vi "PolRaspPiData.vi"(8 "error in (no error)":errorcluster, 11 "VISA Sesssion In":refnum<visa-resource-name>="ASRL6::INSTR") -> (0 "error out":errorcluster, 2 "output array":string[](array[string]), 3 "VISA Sesssion Out":refnum<visa-resource-name>)   [LabVIEW 2019]
panel:
  # "The intention of this is to connect to a raspberry pi and ping for data with either 'Ping' or a number.\nThe intention of this structure is to establish modbus communication. The cRIO cannot acheive this for some reason.\nThe raspPi will monitor the furnace and heatrope data.\nIt will eventually set the furnace setpoint too (later down the line).\n\nThis assumes the serial channel has already been opened"
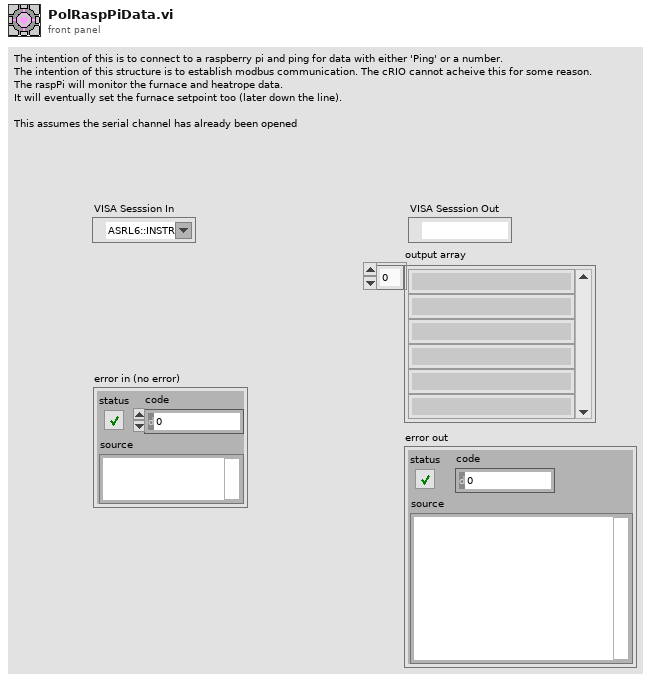
[diagram p1: front panel]
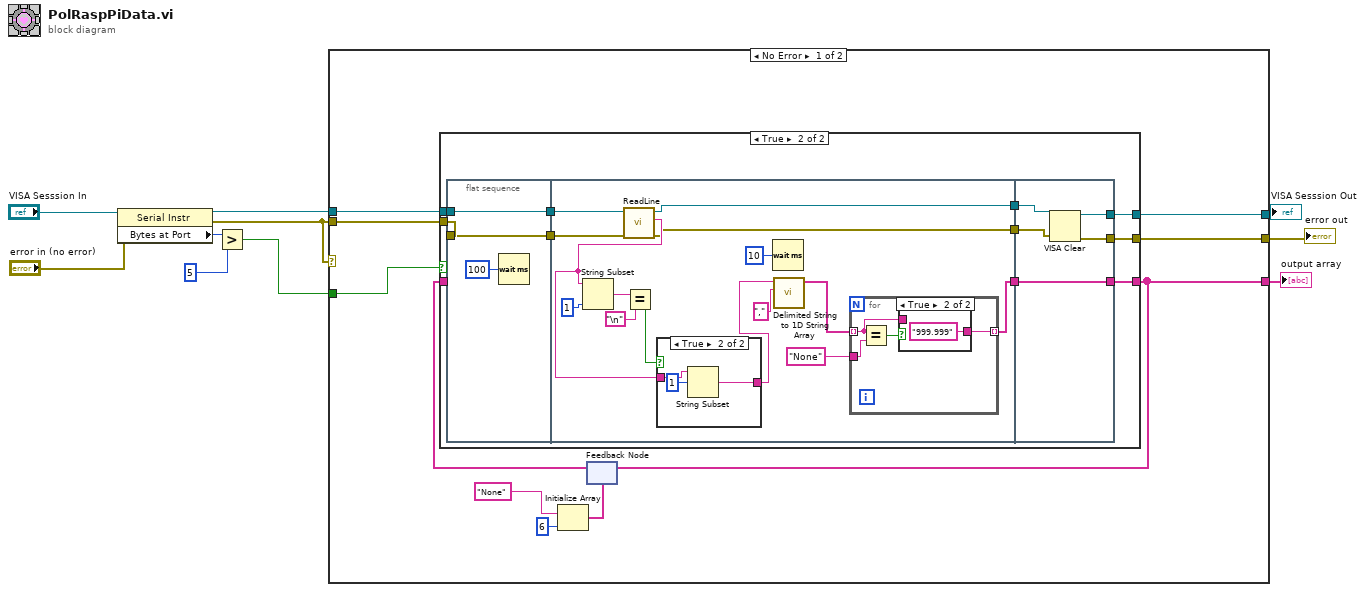
[diagram p0: block diagram]
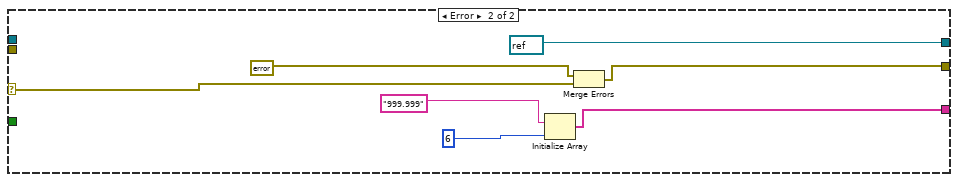
[diagram p5: hidden frame]
diagram:
  n1 = property class="Serial Instr"(reference="VISA Sesssion In", error in="error in (no error)") -> (reference out=w7:refnum<visa-resource-name>, error out=w1:errorcluster, "Bytes at Port"=w9:u32)
  n2 = Greater?(x=w9, y=u32 5) -> (0:w6:bool)
  n3 = case shown="No Error" w1 {
    selector: w1 -> [_ w69]
    tunnel: w7 -> [w20 _]
    tunnel: w1 -> [w19 _]
    tunnel: w6 -> [w18 _]
    tunnel: [w13 w70] -> w4
    tunnel: [w12 w67] -> w3
    tunnel: [w11 refnum<visa-resource-name> refnum ("VISA Sesssion Out")] -> w2
    frame No Error {
      n4 = Initialize Array("None", 6 ("dimension size")) -> (w14:string[])
      n5 = feedback #1(w14) -> (w17:string[])
      n6 = case shown="True" w18 {
        tunnel: [w21 w33] -> w13
        tunnel: w20 -> [w22 w32]
        tunnel: w19 -> [w23 w31]
        tunnel: [w23 w28] -> w12
        tunnel: [w22 w27] -> w11
        tunnel: w17 -> [w21 _]
        frame False {
        }
        frame True {
          n7 = flat-sequence {
            tunnel: w31 -> [w35]
            tunnel: w32 -> [w36]
            tunnel: [w36] -> w30
            tunnel: [w35] -> w29
            tunnel: w30 -> [w50]
            tunnel: w29 -> [w49]
            tunnel: [w37] -> w26
            tunnel: [w42] -> w25
            tunnel: [w41] -> w24
            tunnel: [w62] -> w27
            tunnel: [w63] -> w28
            tunnel: [w66] -> w33
            tunnel: w26 -> [w66]
            tunnel: w25 -> [w65]
            tunnel: w24 -> [w64]
            frame #0 {
              n8 = Wait (ms)(milliseconds to wait=u32 100) -> ()  [unwired: 1 out]
            }
            frame #1 {
              n9 = call "ReadLine.vi"("error in (no error)"=w49, "VISA Sesssion In"=w50) -> ("error out"=w42:errorcluster, "Read Line"=w44:string, "VISA Sesssion Out"=w41:refnum<visa-resource-name>)  [unwired: 7 in]
              n10 = String Subset(string=w44, length (rest)=1 ("length (rest)")) -> (substring=w47:string)  [unwired: 1 in]
              n11 = Equal?(x=w47, y="\n") -> (x = y?=w45:bool)
              n12 = case shown="True" w45 {
                tunnel: w44 -> [w58 w61]
                tunnel: [w58 w59] -> w43
                frame False {
                }
                frame True {
                  n13 = String Subset(string=w61, offset (0)=1) -> (substring=w59:string)  [unwired: 1 in]
                }
              }
              n14 = Wait (ms)(milliseconds to wait=u32 10) -> ()  [unwired: 1 out]
              n15 = call <vilib>:"Delimited String to 1D String Array.vi"("delimiter"=",", "delimited string"=w43) -> ("string array"=w39:string[])  [unwired: 9 in]
              n16 = for {
                tunnel: w39 -> [w53] mode=indexing
                tunnel: "None" ("y") -> [w54]
                tunnel: [w52] -> w37 mode=indexing
                n17 = Equal?(x=w53, y=w54) -> (x = y?=w55:bool)
                n18 = case shown="True" w55 {
                  tunnel: w53 -> [w56 _]
                  tunnel: [w56 "999.999" ("y")] -> w52
                  frame False {
                  }
                  frame True {
                  }
                }
              }
            }
            frame #2 {
              n19 = VISA Clear(VISA resource name=w64, error in (no error)=w65) -> (VISA resource name out=w62:refnum<visa-resource-name>, error out=w63:errorcluster)
            }
          }
        }
      }
      n20 = feedback-in #1(w13) -> ()
    }
    frame Error {
      n21 = Initialize Array("999.999", 6 ("dimension size")) -> (w70:string[])
      n22 = Merge Errors(errorcluster {"status"=TRUE, "code"=0, "source"="Process failed due to earlier errors"} ("error out"), w69) -> (w67:errorcluster)
    }
  }
  "output array" <- w4
  "VISA Sesssion Out" <- w2
  "error out" <- w3
